vi "ProcessMsg.vi"(7 "User":cluster{"pass":string, "User":string}={"pass"="password", "User"="password"}, 8 "Error In":errorcluster, 9 "MessageIn":string, 10 "ServerStatus":T2(ring)=enum."Open Listener", 11 "Auth Status":T1(ring)) -> (0 "Error Out":errorcluster, 1 "MessageOut":string, 2 "ServerStatus out":T2(ring)=enum."Open Listener", 3 "Auth Status Out":T1(ring))   [LabVIEW 2014]
panel:
  out "PasswordIn":string
  out "Username In":string
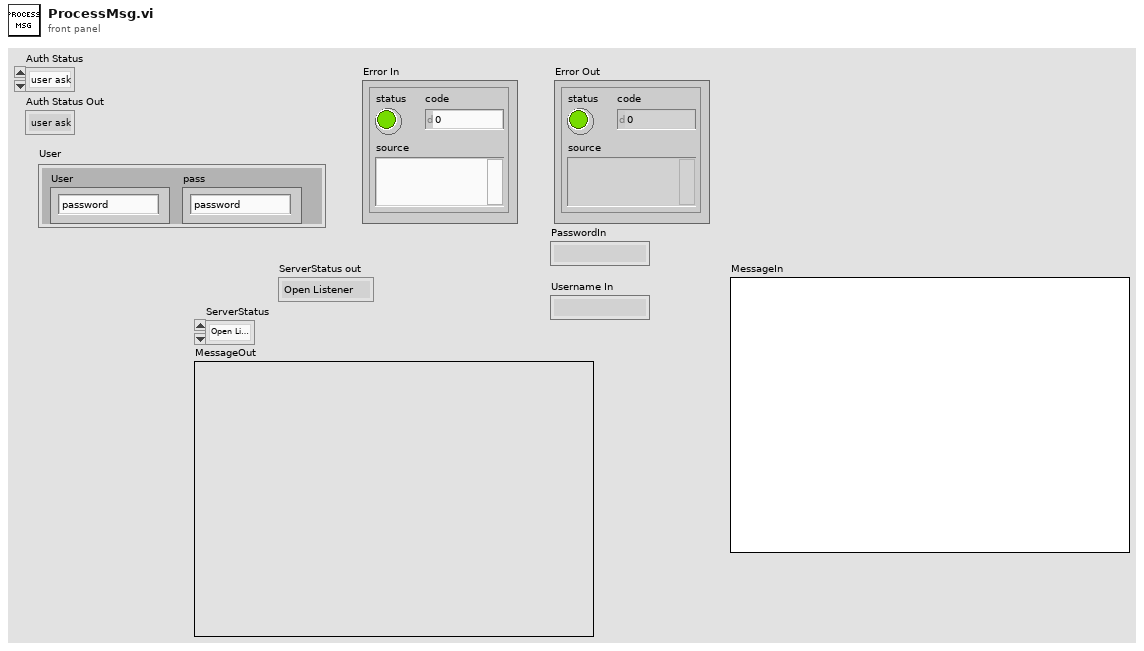
[diagram p1: front panel]
types:
  T1 = enum16{"user ask", "user", "pass ask", "pass", "auth"}
  T2 = enum16{"Poll", "Open Listener", "Generate Certificate", "Wait for Client", "Open SSL Steram", "Read from SSL Stream", "Write Data to SSL Steram", "Close Connection", "Ask Username", "Ask Password", "Parse"}
  T3 = enum16{"Poll", "Open Listener", "Generate Certificate", "Wait for Client", "Open SSL Steram", "Read from SSL Stream", "Write Data to SSL Steram", "Close Connection"}
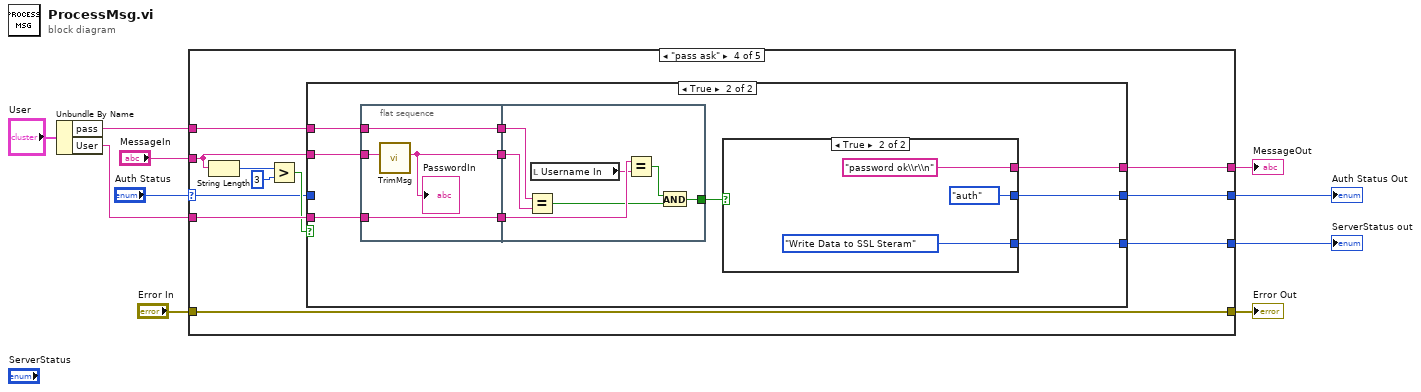
[diagram p0: block diagram]
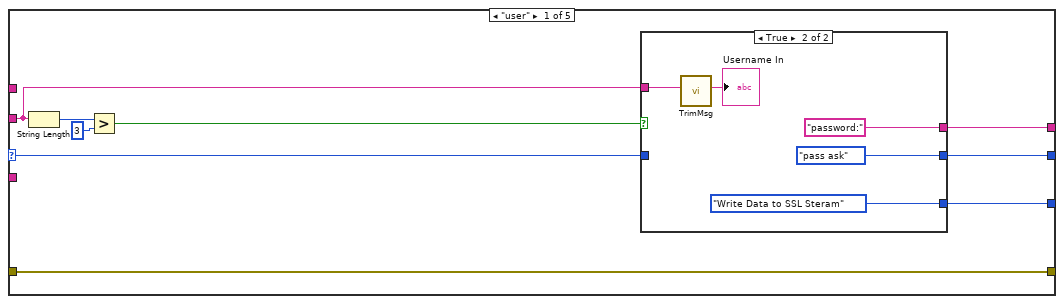
[diagram p2: hidden frame]
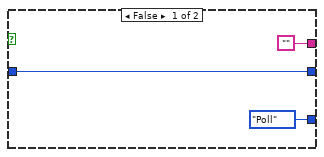
[diagram p3: hidden frame]
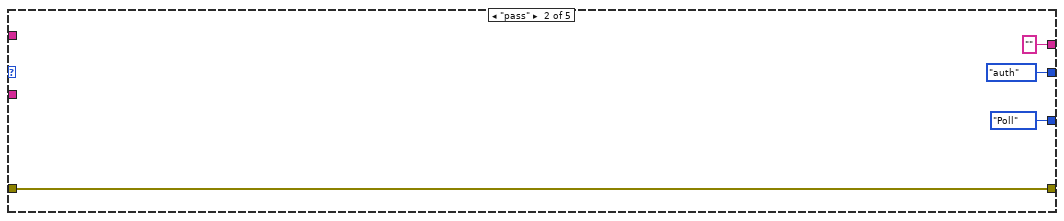
[diagram p4: hidden frame]
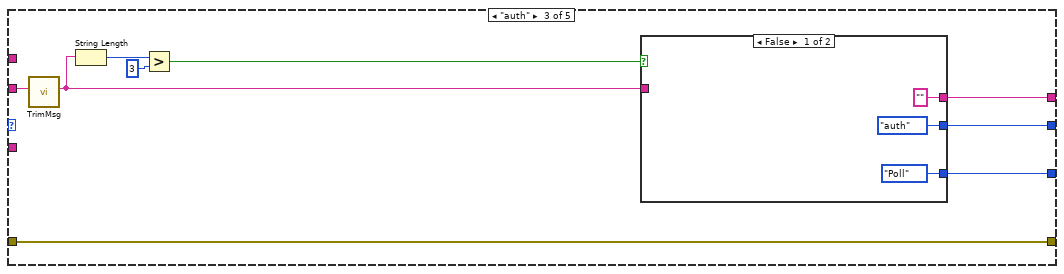
[diagram p5: hidden frame]
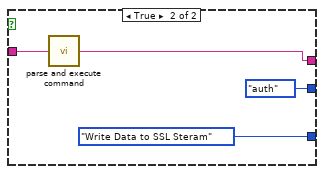
[diagram p6: hidden frame]
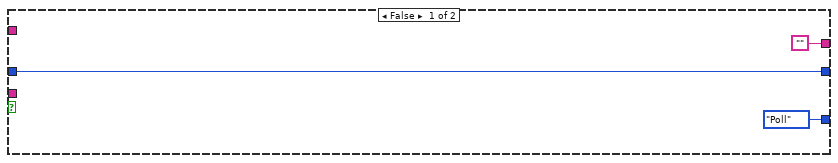
[diagram p7: hidden frame]
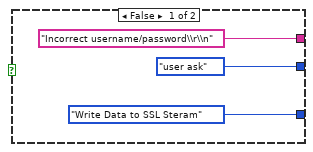
[diagram p8: hidden frame]
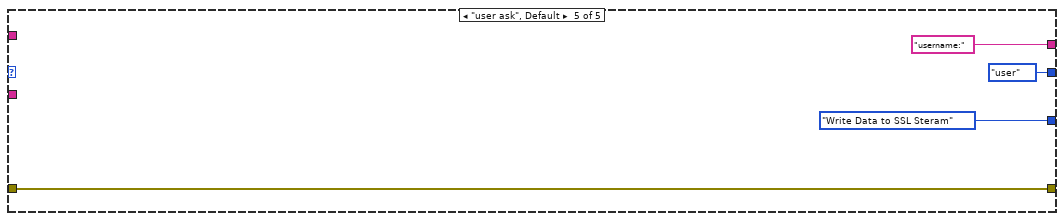
[diagram p9: hidden frame]
diagram:
  n1 = Unbundle By Name("User") -> ("pass"=w2:string, "User"=w1:string)
  n2 = case shown="\"pass ask\"" "Auth Status" {
    selector: "Auth Status" -> [w12 _ _ w49 _]
    tunnel: [w19 T1."auth" w33 w55 T1."user"] -> w9
    tunnel: [w18 "" w39 w56 "username:"] -> w8
    tunnel: [w17 T3."Poll" w32 w54 T3."Write Data to SSL Steram"] -> w7
    tunnel: "Error In" -> [w16 w29 w40 w53 w89]
    tunnel: [w16 w29 w40 w53 w89] -> w5
    tunnel: "MessageIn" -> [w11 _ w38 w48 _]
    tunnel: w1 -> [_ _ _ w58 _]
    tunnel: w2 -> [_ _ _ w57 _]
    frame "user" {
      n3 = String Length(string=w11) -> (length=w15:i32)
      n4 = Greater?(x=w15, y=3) -> (0:w13:bool)
      n5 = case shown="True" w13 {
        tunnel: [w22 T1."pass ask"] -> w19
        tunnel: ["" "password:"] -> w18
        tunnel: [T3."Poll" T3."Write Data to SSL Steram"] -> w17
        tunnel: w12 -> [w22 _]
        tunnel: w11 -> [_ w23]
        frame False {
        }
        frame True {
          n6 = call <userlib>:"TrimMsg.vi"("Message"=w23) -> ("Msg"=→"Username In":string)  [unwired: 10 in]
        }
      }
    }
    frame "pass" {
    }
    frame "auth" {
      n7 = call <userlib>:"TrimMsg.vi"("Message"=w38) -> ("Msg"=w37:string)  [unwired: 10 in]
      n8 = String Length(string=w37) -> (length=w36:i32)
      n9 = Greater?(x=w36, y=3) -> (0:w34:bool)
      n10 = case shown="False" w34 {
        tunnel: ["" ("Python Return String") w47] -> w39
        tunnel: w37 -> [_ w46]
        tunnel: [T1."auth" T1."auth"] -> w33
        tunnel: [T3."Poll" T3."Write Data to SSL Steram"] -> w32
        frame False {
        }
        frame True {
          n11 = call <userlib>:"parse and execute command.vi"("Python Command"=w46) -> ("Python Return String"=w47:string)
        }
      }
    }
    frame "pass ask" {
      n12 = String Length(string=w48) -> (length=w52:i32)
      n13 = Greater?(x=w52, y=3) -> (0:w50:bool)
      n14 = case shown="True" w50 {
        tunnel: w58 -> [_ w71]
        tunnel: w57 -> [_ w70]
        tunnel: ["" w68] -> w56
        tunnel: [w60 w67] -> w55
        tunnel: [T3."Poll" w66] -> w54
        tunnel: w49 -> [w60 _]
        tunnel: w48 -> [_ w63]
        frame False {
        }
        frame True {
          n15 = flat-sequence {
            tunnel: w70 -> [w74]
            tunnel: w71 -> [w75]
            tunnel: [w75] -> w65
            tunnel: [w74] -> w64
            tunnel: w63 -> [w73]
            tunnel: [w72] -> w62
            tunnel: [w77] -> w69
            tunnel: w65 -> [w82]
            tunnel: w64 -> [w81]
            tunnel: w62 -> [w76]
            frame #0 {
              n16 = call <userlib>:"TrimMsg.vi"("Message"=w73) -> ("Msg"=w72:string)  [unwired: 10 in]
              "PasswordIn" <- w72
            }
            frame #1 {
              n17 = Equal?(x=w81, y=w76) -> (x = y?=w78:bool)
              n18 = local read "Username In"() -> (w80:string)
              n19 = Equal?(x=w82, y=w80) -> (x = y?=w79:bool)
              n20 = And(x=w79, y=w78) -> (x .and. y?=w77:bool)
            }
          }
          n21 = case shown="True" w69 {
            tunnel: ["Incorrect username/password\\r\\n" "password ok\\r\\n"] -> w68
            tunnel: [T1."user ask" T1."auth"] -> w67
            tunnel: [T3."Write Data to SSL Steram" T3."Write Data to SSL Steram"] -> w66
            frame False {
            }
            frame True {
            }
          }
        }
      }
    }
    frame "user ask", Default {
    }
  }
  "MessageOut" <- w8
  "ServerStatus out" <- w7
  "Error Out" <- w5
  "Auth Status Out" <- w9
